vi "GetAllUsers.vi"(8 "error in (no error)":errorcluster, 9 "Sequence Context In":refnum<k7>) -> (0 "Array":string[](array[string]), 2 "error out":errorcluster, 3 "Sequence Context Out":refnum<k7>)   [LabVIEW 2020]
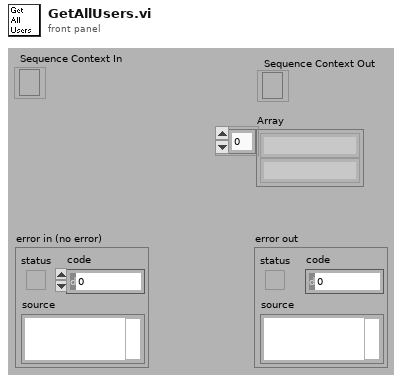
[diagram p1: front panel]
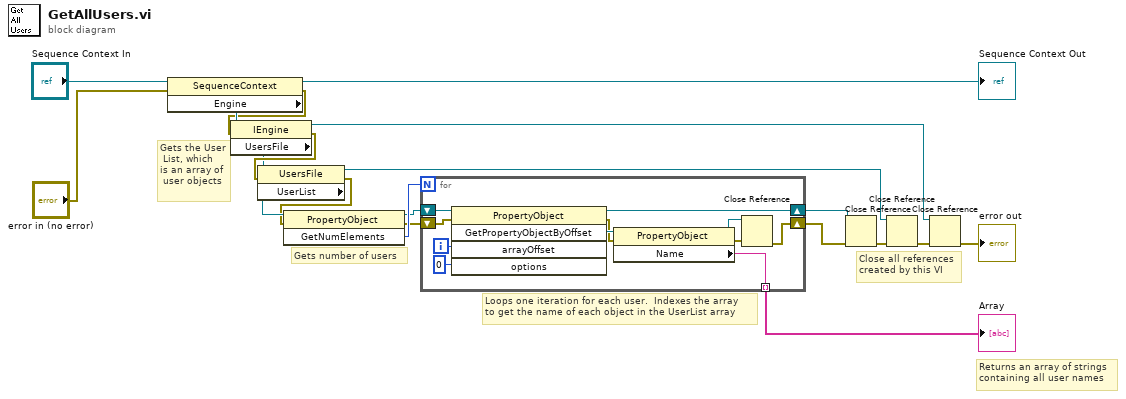
[diagram p0: block diagram]
diagram:
  # "Returns an array of strings\ncontaining all user names"
  # "Close all references\ncreated by this VI"
  # "Loops one iteration for each user.  Indexes the array\nto get the name of each object in the UserList array"
  # "Gets number of users"
  # "Gets the User\n List, which\nis an array of\n user objects"
  n1 = property class="SequenceContext"(reference="Sequence Context In", error in="error in (no error)") -> (reference out=→"Sequence Context Out":refnum<k7>, error out=w4:errorcluster, "Engine"=w6:refnum<k7>)
  n2 = property class="IEngine"(reference=w6, error in=w4) -> (reference out=w7:refnum<k7>, error out=w20:errorcluster, "UsersFile"=w19:refnum<k7>)
  n3 = property class="UsersFile"(reference=w19, error in=w20) -> (reference out=w9:refnum<k7>, error out=w17:errorcluster, "UserList"=w18:refnum<k7>)
  n4 = invoke class="PropertyObject" method="GetNumElements"(reference=w18, error in=w17) -> (reference out=w15:refnum<k7>, error out=w13:errorcluster, "GetNumElements"=w16:i32)  [unwired: 1 in]
  n5 = for {
    N: w16 -> [_]
    tunnel: [w24] -> w14 mode=indexing
    shift-right: [w23] -> w12
    shift-left: w13 -> [w21]
    shift-right: [w22] -> w11
    shift-left: w15 -> [w31]
    i -> [w30]
    n6 = invoke class="PropertyObject" method="GetPropertyObjectByOffset"(reference=w31, error in=w21, "arrayOffset"=w30, "options"=0) -> (reference out=w22:refnum<k7>, error out=w27:errorcluster, "GetPropertyObjectByOffset"=w28:refnum<k7>)  [unwired: 1 in, 2 out]
    n7 = property class="PropertyObject"(reference=w28, error in=w27) -> (reference out=w26:refnum<k7>, error out=w25:errorcluster, "Name"=w24:string)
    n8 = Close Reference(reference=w26, error in (no error)=w25) -> (error out=w23:errorcluster)
  }
  "Array" <- w14
  n9 = Close Reference(reference=w11, error in (no error)=w12) -> (error out=w10:errorcluster)
  n10 = Close Reference(reference=w9, error in (no error)=w10) -> (error out=w8:errorcluster)
  n11 = Close Reference(reference=w7, error in (no error)=w8) -> (error out=→"error out":errorcluster)
